vi "Save inspection prog  to IPF.vi"(0 "Programming Data in":T12, 1 "Set Initial flag":bool, 5 "APG Config":T13, 7 "data in":T1, 11 "error in":errorcluster) -> (4 "Programming Data out":T12, 8 "data out":T1, 15 "error out":errorcluster)   [LabVIEW 2013, in "Manipulate IPF.lvlib"]
uses:
  Manipulate IPF.lvlib
  3013/code/Modules/GUI/GUI_5/subPanels/edit/type_def/data.ctl
  3013/code/Modules/Configuration/type_def/Scan Params.ctl
  3013/code/Modules/Configuration/type_def/Profile Resolution.ctl
  3013/code/Modules/Preprocess Data/type_def/direction.ctl
  3013/code/Modules/Inspection/Data/Panel_class/type_def/Config File data.ctl
  3013/code/Modules/Inspection/type_def/Pos and Rot.ctl
  3013/code/Modules/Inspection/Data/PCB_class/type_def/PCB Params.ctl
  3013/code/Modules/Inspection/Data/Panel_class/type_def/BarCode Params.ctl
  3013/code/Modules/Barcode Reader/type_def/id.ctl
  3013/code/Modules/Inspection/Data/Panel_class/type_def/inspection data.ctl
  3013/code/Modules/Inspection/type_def/Range Limits.ctl
  Settings/type_def/APG Config.ctl
  type_def/files.ctl
  Pack Data/type_def/file types.ctl
  Pack Data/Pack Files.lvlib
  3013/code/Modules/Inspection/Inspection.lvlib
  3013/code/Modules/Inspection/Data/PCB_class/PCB.lvclass
  3013/code/Modules/Barcode Reader/Barcode Reader.lvlib
  3013/code/Modules/Inspection/Data/Panel_class/Panel.lvclass
  3013/code/Modules/Configuration/Config.lvlib
  3013/code/Modules/Preprocess Data/PreProcess.lvlib
  3013/code/Modules/GUI/GUI_5/subPanels/edit/edit.lvlib
  Settings/APG_settings.lvlib
  a3Di APG.lvlib
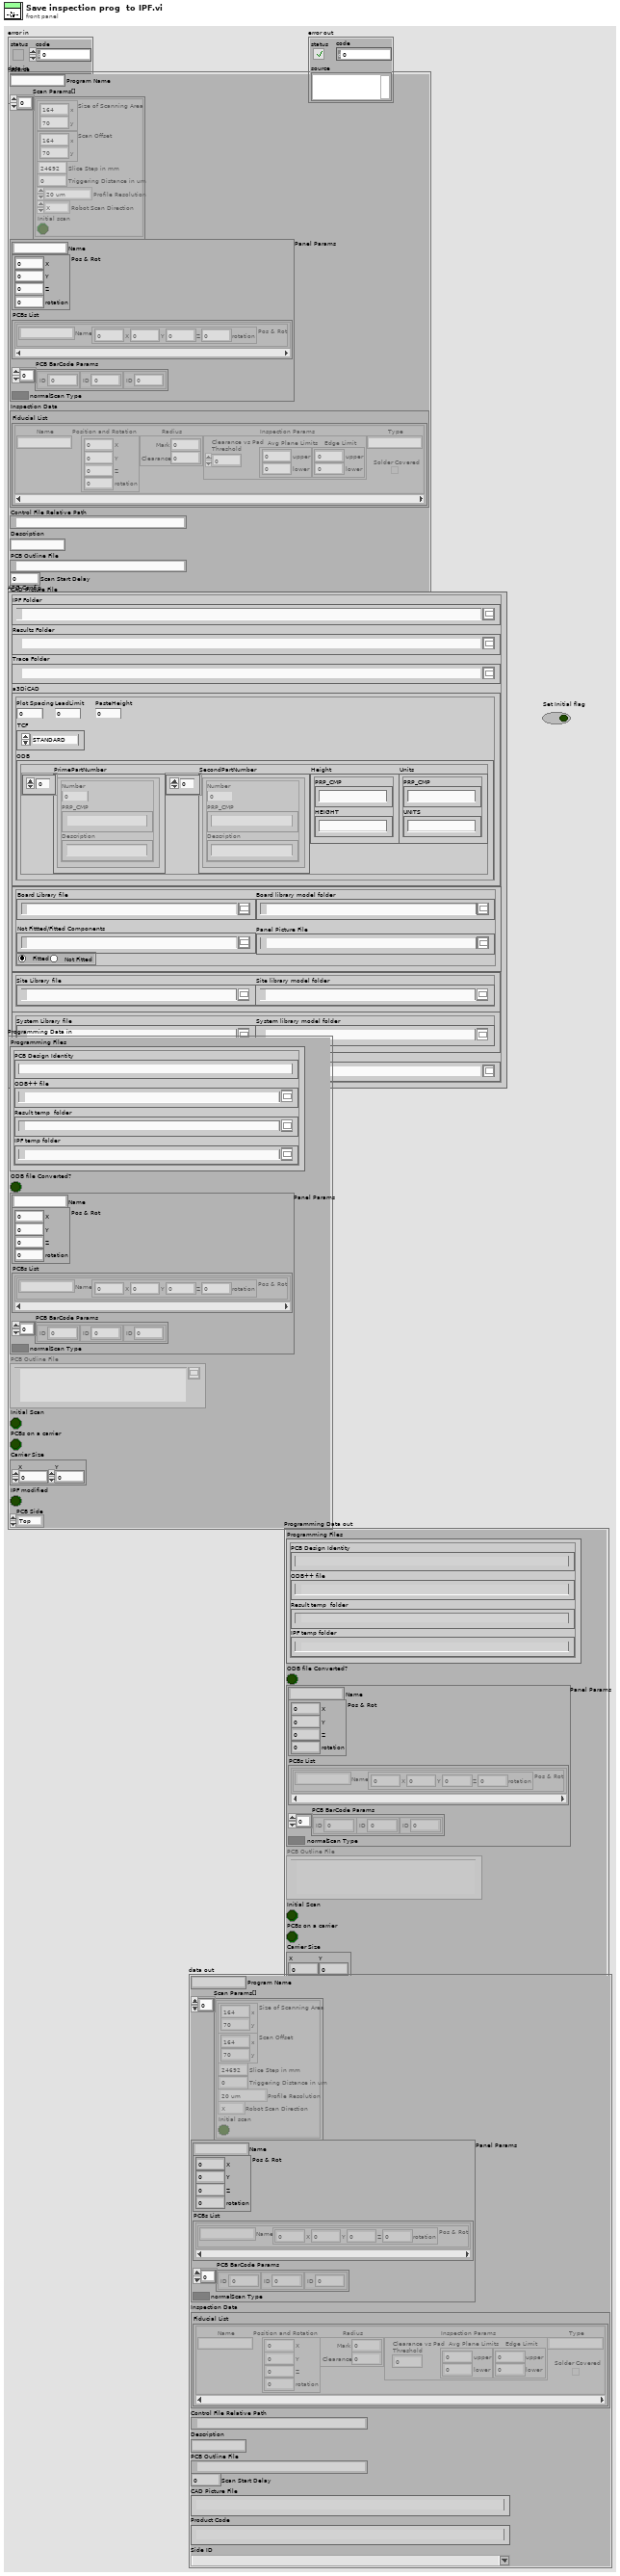
[diagram p1: front panel]
types:
  T1 = typedef "GUI.lvlib/subPanel.lvlib/edit.lvlib/data.ctl" = cluster{"Program Name":string, "Scan Params[]":T2[], "Panel Params":T5, "Inspection Data":T10, "Control File Relative Path":path, "Description":string, "PCB Outline File":path, "Scan Start Delay":dbl, "CAD Picture File":string, "Product Code":string, "Side ID":string}
  T2 = typedef "Config.lvlib/Scan Params.ctl" = cluster{"Size of Scanning Area":cluster{"x":dbl, "y":dbl}, "Scan Offset":cluster{"x":dbl, "y":dbl}, "Slice Step in mm":dbl, "Triggering Distance in mm":dbl, "Triggering Distance in um":dbl, "Profile Resolution":T3, "Version":string, "Robot Scan Direction":T4, "Initial scan":bool}
  T3 = typedef "Config.lvlib/Profile Resolution.ctl" = enum8{"20 um", "40 um"}
  T4 = typedef "PreProcess.lvlib/direction.ctl" = enum8{"X", "Y"}
  T5 = typedef "Inspection.lvlib/Panel.lvclass/Config File data.ctl" = cluster{"Name":string, "Pos & Rot":T6, "PCBs List":cluster{"PCB Params":T7}[], "PCB BarCode Params":T8[], "Scan Type":bool}
  T6 = typedef "Inspection.lvlib/Pos and Rot.ctl" = cluster{"X":dbl, "Y":dbl, "Z":dbl, "rotation":dbl}
  T7 = typedef "Inspection.lvlib/PCB.lvclass/PCB Params.ctl" = cluster{"Name":string, "Pos & Rot":T6}
  T8 = typedef "Inspection.lvlib/Panel.lvclass/BarCode Params.ctl" = cluster{"ID":T9}
  T9 = typedef "Barcode Reader.lvlib/id.ctl" = u8
  T10 = typedef "Inspection.lvlib/Panel.lvclass/inspection data.ctl" = cluster{"Fiducial List":cluster{"Name":string, "Position and Rotation":T6, "Radius":cluster{"Mark":dbl, "Clearance":dbl}, "Inspection Params":cluster{"Clearance vs Pad\nThreshold":dbl, "Avg Plane Limits":T11, "Edge Limit":T11}, "Type":string, "Solder Covered":bool}[]}
  T11 = typedef "Inspection.lvlib/Range Limits.ctl" = cluster{"upper":sgl, "lower":sgl}
  T12 = typedef "a3Di APG.lvlib/files.ctl" = cluster{"Programming Files":cluster{"PCB Design Identity":string, "ODB++ file":path, "Result temp  folder":path, "IPF temp folder":path}, "ODB file Converted?":bool, "Panel Params":T5, "PCB Outline File":path, "Initial Scan":bool, "PCBs on a carrier":bool, "Carrier Size":cluster{"X":dbl, "Y":dbl}, "IPF modified":bool, "PCB Side":enum16{"Top", "Bottom"}}
  T13 = typedef "APG_settings.lvlib/APG Config.ctl" = cluster{"IPF Folder":path, "Results Folder":path, "Trace Folder":path, "a3DiCAD":cluster{"Plot Spacing":dbl, "TCF":enum16{"STANDARD", "PASTE", "LEAD"}, "LeadLimit":u32, "a3DiCADDebug":bool, "ODB":cluster{"PrimePartNumber":cluster{"Number":u32, "PRP_CMP":string, "Description":string}[], "SecondPartNumber":cluster{"Number":u32, "PRP_CMP":string, "Description":string}[], "Height":cluster{"PRP_CMP":string, "HEIGHT":string}, "Units":cluster{"PRP_CMP":string, "UNITS":string}}, "PasteHeight":dbl}, "a3DiCADcfg":path, "Board Library":cluster{"Board Library file":path, "Board library model folder":path, "Not Fittted/Fitted Components":path, "Panel Picture File":path, "Components":enum32{"Fitted", "Not Fitted "}}, "Site Library":cluster{"Site Library file":path, "Site library model folder":path}, "System Library":cluster{"System Library file":path, "System library model folder":path}, "ODB++ file":path}
  T14 = typedef "Pack Files.lvlib/file types.ctl" = enum16{"ODB", "TCF", "CAD Outline", "Config", "Inspection Prog", "a3Di-bin", "Results", "CAD Labels", "CAD Pads", "calScan_fid", "calScan_cal-tab", "PCB_SerialNumber", "CAD_Assembly", "Version", "Old Results", "CAD Picture", "Old TCF"}
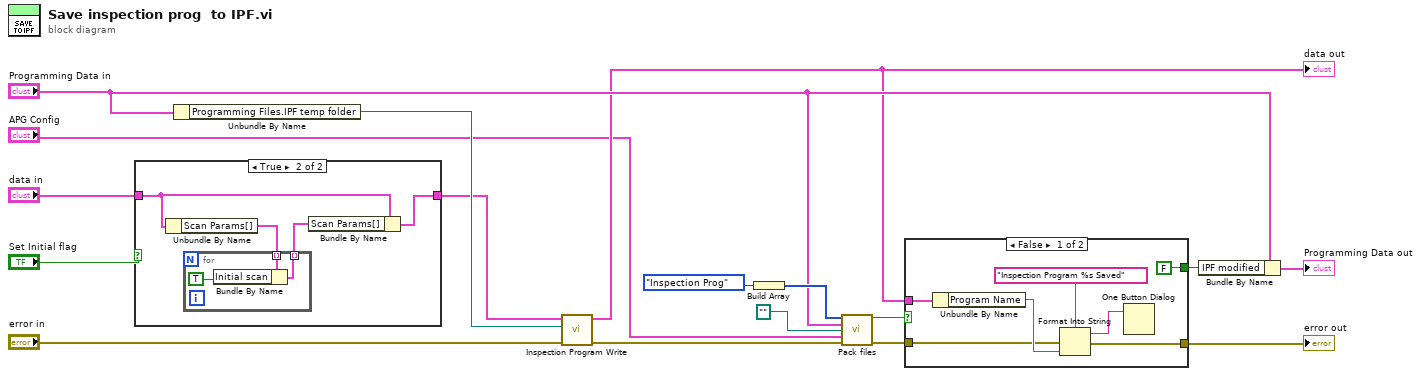
[diagram p0: block diagram]
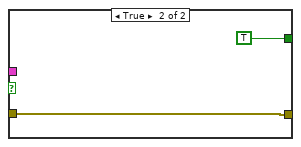
[diagram p3: hidden frame]
diagram:
  n1 = case shown="True" "Set Initial flag" {
    tunnel: [w18 w22] -> w3
    tunnel: "data in" -> [w18 w19]
    frame False {
    }
    frame True {
      n2 = Unbundle By Name(w19) -> ("Scan Params[]"=w21:T2[])
      n3 = for {
        tunnel: w21 -> [w24] mode=indexing
        tunnel: [w23] -> w20 mode=indexing
        n4 = Bundle By Name(cluster=w24, "Initial scan"=TRUE ("Initial Scan")) -> (w23:T2)
      }
      n5 = Bundle By Name(cluster=w19, "Scan Params[]"=w20) -> (w22:T1)
    }
  }
  n6 = Unbundle By Name("Programming Data in") -> ("Programming Files.IPF temp folder"=w17:path)
  n7 = call "Inspection Program Write.vi"("error in (no error)"="error in", "IPF Folder"=w17, "data in"=w3) -> ("error out"=w12:errorcluster, "data out"=w7:T1)  [unwired: 7 in]
  "data out" <- w7
  n8 = Build Array(file_types."Inspection Prog" ("Descriptions")) -> (w13:T14[])
  n9 = call "Pack files.vi"("File type[]"=w13, "Programming Data In"="Programming Data in", "TCF/CAD Picture file"=path "", "APG Config"="APG Config", "error in (no error)"=w12) -> ("Error detected"=w2:bool, "error out"=w1:errorcluster)  [unwired: 9 in]
  n10 = case shown="False" w2 {
    tunnel: [w32 w33] -> w9
    tunnel: [FALSE ("IPF saved") TRUE ("IPF saved")] -> w14
    tunnel: w7 -> [w28 _]
    tunnel: w1 -> [w26 w33]
    frame False {
      n11 = Unbundle By Name(w28) -> ("Program Name"=w27:string)
      n12 = Format Into String(format string="Inspection Program %s Saved", error in=w26, w27) -> (resulting string=w31:string, error out=w32:errorcluster)  [unwired: 1 in]
      n13 = One Button Dialog(message=w31) -> ()  [unwired: 1 in, 1 out]
    }
    frame True {
    }
  }
  "error out" <- w9
  n14 = Bundle By Name(cluster="Programming Data in", "IPF modified"=w14) -> (→"Programming Data out":T12)
